vi "Read Skipped RUNs.vi"(8 "error in (no error)":errorcluster, 11 "Run Block in":refnum<class "Run Block.lvclass">) -> (0 "error out":errorcluster, 2 "Skipped RUNs":refnum<class "Schedule.lvclass">, 3 "Run Block out":refnum<class "Run Block.lvclass">)   [LabVIEW 2020, in "Run Utilities.lvlib" / "Run Block.lvclass"]
uses:
  Run Block.lvclass
  Schedule/Schedule.lvclass
  Run Block.lvclass/Run Block.ctl
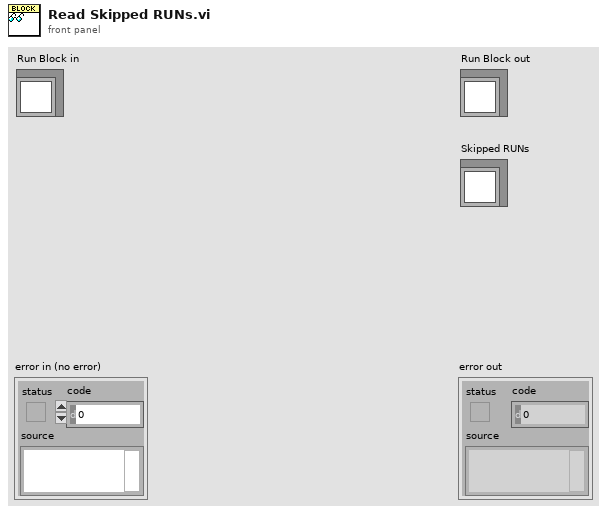
[diagram p1: front panel]
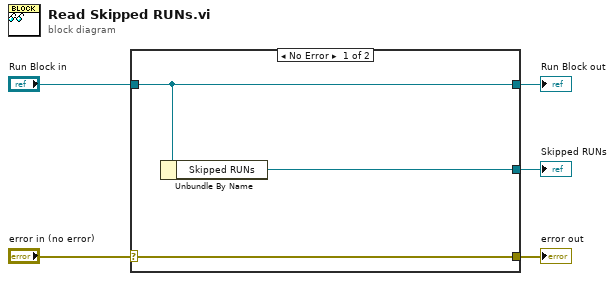
[diagram p0: block diagram]
diagram:
  n1 = case shown="No Error" "error in (no error)" {
    selector: "error in (no error)" -> [w8 w9]
    tunnel: [w8 w9] -> w4
    tunnel: [w7 w10] -> w2
    tunnel: "Run Block in" -> [w7 w10]
    tunnel: [w6 _] -> w1
    frame No Error {
      n2 = Unbundle By Name(w7) -> ("Skipped RUNs"=w6:refnum<class "Schedule.lvclass">)
    }
    frame Error {
    }
  }
  "error out" <- w4
  "Run Block out" <- w2
  "Skipped RUNs" <- w1
